vi "sudoku.vi"() -> ()   [LabVIEW 2017]
uses:
  <vilib>/Analysis/Matrix/Datatypes/RealMatrix.ctl
  <vilib>/Analysis/Matrix/Numeric/Conversions/Array To Matrix - RA.vi
  <vilib>/Analysis/Matrix/Numeric/Multiply/Multiply - RM,RM.vi
  <vilib>/Analysis/Matrix/NI_Matrix.lvlib
panel:
  out "Gauge":dbl(knob) scale=0.0..10.0
  in  "Slide 2":dbl(slide) scale=0.0..10.0
  in  "Slide":dbl(slide) scale=0.0..10.0
  in  "Boolean 2":bool
  in  "Boolean":bool
  out "element 2":dbl
  out "Real Matrix (Column Vector) 2":T1
  out "Real Matrix (Column Vector)":T1
  out "A * B":T1
  out "output array 2":dbl[][](array[numeric])
  in  "NumSteps":i32
  out "solution":dbl[][](array[numeric])
  out "x = y?":bool
  out "element":dbl
  out "columns":dbl[](array[numeric])
  out "rows":dbl[](array[numeric])
  out "sqare":dbl[][](array[numeric])
  out "output array":dbl[][](array[numeric])
  in  "Array 9":dbl[][](array[numeric])
  in  "Array 8":dbl[][](array[numeric])
  in  "Array 7":dbl[][](array[numeric])
  in  "Array 6":dbl[][](array[numeric])
  in  "Array 5":dbl[][](array[numeric])
  in  "Array 4":dbl[][](array[numeric])
  in  "Array 3":dbl[][](array[numeric])
  in  "Array 2":dbl[][](array[numeric])
  in  "Array":dbl[][](array[numeric])
  # "Toto pridal Master"
  # "Toto je sprava z Develu."
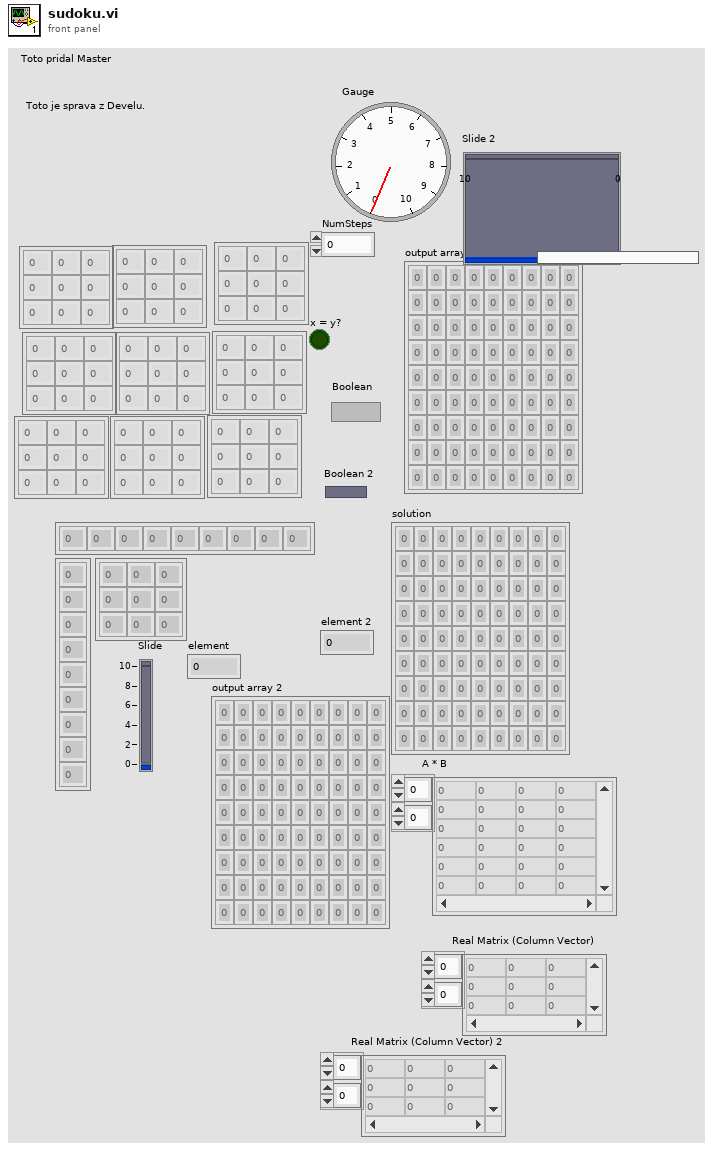
[diagram p1: front panel]
types:
  T1 = typedef "NI_Matrix.lvlib/RealMatrix.ctl" = dbl[][]
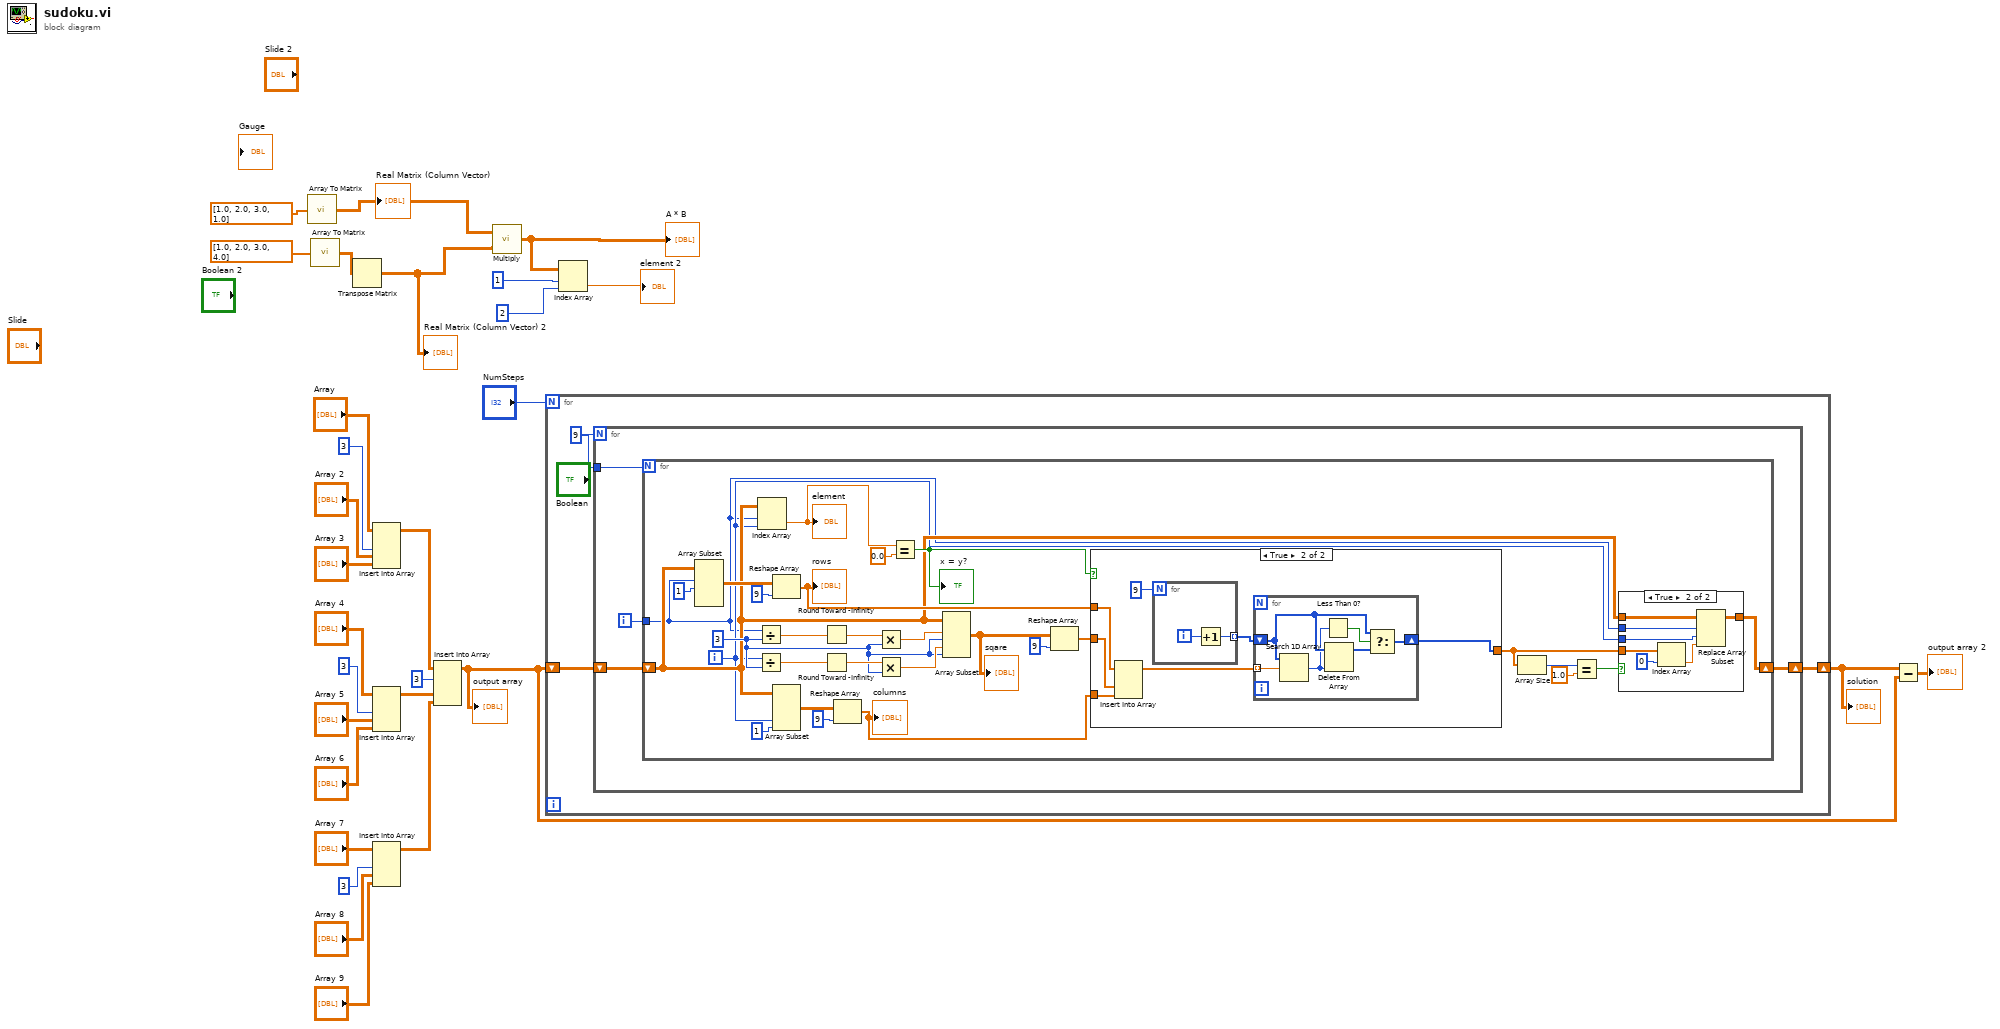
[diagram p0: block diagram]
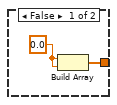
[diagram p3: hidden frame]
diagram:
  n1 = call-poly <vilib>:"Array To Matrix.vi"("Real 1D Array"=dbl[] [1.0, 2.0, 3.0, 1.0]) -> ("Real Matrix (Column Vector)"=w7:T1)
  "Real Matrix (Column Vector)" <- w7
  n2 = call-poly <vilib>:"Array To Matrix.vi"("Real 1D Array"=dbl[] [1.0, 2.0, 3.0, 4.0]) -> ("Real Matrix (Column Vector)"=w6:T1)
  n3 = Transpose Matrix(1:w6) -> (0:w5:T1)
  "Real Matrix (Column Vector) 2" <- w5
  n4 = Insert Into Array(array="Array", index (col)=3 ("disabled index (col)"), new element #1="Array 2", new element #2="Array 3") -> (w14:dbl[][])  [unwired: 1 in]
  n5 = Insert Into Array(array="Array 4", index (col)=3 ("disabled index (col)"), new element #1="Array 5", new element #2="Array 6") -> (w15:dbl[][])  [unwired: 1 in]
  n6 = Insert Into Array(array="Array 7", index (col)=3 ("disabled index (col)"), new element #1="Array 8", new element #2="Array 9") -> (w16:dbl[][])  [unwired: 1 in]
  n7 = Insert Into Array(array=w14, index (row)=3, new element #1=w15, new element #2=w16) -> (w12:dbl[][])  [unwired: 1 in]
  "output array" <- w12
  n8 = call-poly <vilib>:"Multiply.vi"("Real Matrix B"=w5, "Real Matrix A"=w7) -> ("A * B"=w4:T1)
  "A * B" <- w4
  n9 = for {
    N: "NumSteps" -> [_]
    shift-right: [w32] -> w11
    shift-left: w12 -> [w31]
    w30 = 9
    n10 = for {
      N: w30 -> [_]
      shift-right: [w36] -> w32
      shift-left: w31 -> [w35]
      tunnel: w30 -> [w33]
      i -> [w34]
      n11 = for {
        N: w33 -> [_]
        shift-right: [w41] -> w36
        shift-left: w35 -> [w39]
        tunnel: w34 -> [w37]
        i -> [w38]
        w54 = 3 ("length")
        n12 = Array Subset(array=w39, index (row)=w37, length (row)=1 ("length")) -> (w47:dbl[][])  [unwired: 2 in]
        n13 = Divide(x=w37, y=w54) -> (x/y=w58:dbl)
        n14 = Divide(x=w38, y=w54) -> (x/y=w57:dbl)
        n15 = Index Array(array=w39, index (row)=w37, index (col)=w38) -> (element=w53:dbl)
        "element" <- w53
        n16 = Reshape Array(w47, 9 ("dimension size")) -> (w50:dbl[])
        "rows" <- w50
        n17 = Array Subset(array=w39, index (col)=w38, length (col)=1 ("length")) -> (w59:dbl[][])  [unwired: 2 in]
        n18 = Round Toward -Infinity(1:w58) -> (0:w55:dbl)
        n19 = Round Toward -Infinity(1:w57) -> (0:w56:dbl)
        n20 = Reshape Array(w59, 9 ("dimension size")) -> (w45:dbl[])
        "columns" <- w45
        n21 = Multiply(x=w55, y=w54) -> (x*y=w65:dbl)
        n22 = Multiply(x=w56, y=w54) -> (x*y=w64:dbl)
        n23 = Equal?(x=w53, y=0.0) -> (x = y?=w51:bool)
        "x = y?" <- w51
        n24 = Array Subset(array=w39, index (row)=w65, length (row)=w54, index (col)=w64, length (col)=w54) -> (w49:dbl[][])
        "sqare" <- w49
        n25 = Reshape Array(w49, 9 ("dimension size")) -> (w46:dbl[])
        n26 = case shown="True" w51 {
          tunnel: w50 -> [_ w78]
          tunnel: [w75 w80] -> w40
          tunnel: w46 -> [_ w76]
          tunnel: w45 -> [_ w77]
          frame False {
            w74 = 0.0 ("element")
            n27 = Build Array(w74, w74) -> (w75:dbl[])
          }
          frame True {
            n28 = Insert Into Array(array=w78, new element #1=w76, new element #2=w77) -> (w79:dbl[])  [unwired: 1 in]
            n29 = for {
              N: 9 -> [_]
              tunnel: [w90] -> w81 mode=indexing
              i -> [w89]
              n30 = Increment(x=w89) -> (x+1=w90:i32)
            }
            n31 = for {
              tunnel: w79 -> [w83] mode=indexing
              shift-right: [w87] -> w80
              shift-left: w81 -> [w85]
              n32 = Search 1D Array(1D array=w85, element=w83) -> (index of element=w84:i32)  [unwired: 1 in]
              n33 = Less Than 0?(x=w84) -> (x < 0?=w88:bool)
              n34 = Delete From Array(array=w85, index=w84) -> (array with subset deleted=w86:i32[])  [unwired: 1 in, 1 out]
              n35 = Select(t=w85, s=w88, f=w86) -> (s? t:f=w87:i32[])
            }
          }
        }
        n36 = Array Size(array=w40) -> (size(s)=w43:i32)
        n37 = Equal?(x=w43, y=1.0) -> (x = y?=w42:bool)
        n38 = case shown="True" w42 {
          tunnel: w39 -> [w66 w73]
          tunnel: [w66 w69] -> w41
          tunnel: w37 -> [_ w72]
          tunnel: w38 -> [_ w68]
          tunnel: w40 -> [_ w71]
          frame False {
          }
          frame True {
            n39 = Index Array(array=w71, index=0) -> (element=w67:dbl)
            n40 = Replace Array Subset(array=w73, new element=w67, index (row)=w72, index (col)=w68) -> (w69:dbl[][])
          }
        }
      }
    }
  }
  "solution" <- w11
  n41 = Index Array(array=w4, index (row)=1, index (col)=2 ("disabled index (col)")) -> (element=→"element 2":dbl)
  n42 = Subtract(x=w11, y=w12) -> (x-y=→"output array 2":dbl[][])
